vi "F Dwf Analog Out Data Info.vi"(7 "pnSamplesMax":i32, 8 "error in (no error)":errorcluster, 9 "pnSamplesMin":i32, 10 "idxChannel":i32, 11 "hdwf":i32) -> (0 "error out":errorcluster, 1 "pnSamplesMin out":i32, 3 "function return":i32, 5 "pnSamplesMax out":i32)   [LabVIEW 2021, in "Olasdwf.lvlib"]
doc: "DWFAPI int FDwfAnalogOutDataInfo(HDWF hdwf, int idxChannel, int *pnSamplesMin, int *pnSamplesMax);"
uses:
  Olasdwf.lvlib
  Windows/System32/dwf.dll
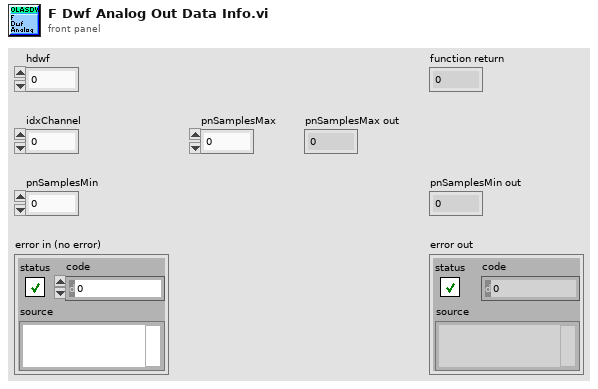
[diagram p1: front panel]
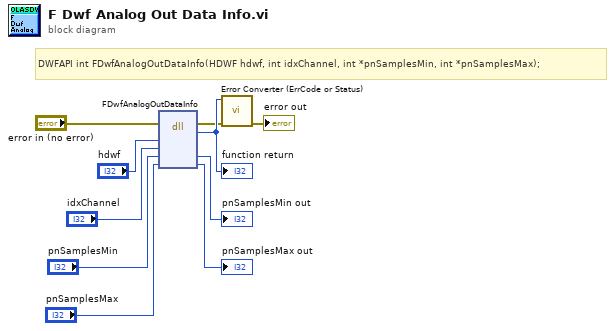
[diagram p0: block diagram]
diagram:
  # "DWFAPI int FDwfAnalogOutDataInfo(HDWF hdwf, int idxChannel, int *pnSamplesMin, int *pnSamplesMax);"
  n1 = dll-call lib="/Windows/System32/dwf.*" fn="FDwfAnalogOutDataInfo"(error in="error in (no error)", "hdwf"="hdwf", "idxChannel"="idxChannel", "pnSamplesMin"="pnSamplesMin", "pnSamplesMax"="pnSamplesMax") -> (error out=w2:errorcluster, w10:i32, "pnSamplesMin"=→"pnSamplesMin out":i32, "pnSamplesMax"=→"pnSamplesMax out":i32)  [unwired: 4 in, 1 out]
  "function return" <- w10
  n2 = call "Error Converter (ErrCode or Status).vi"("error in (no error)"=w2, "error code"=w10) -> ("error out"=→"error out":errorcluster)  [unwired: 9 in]
